vi "Upgrade Firmware (File).vi"(6 "Remote Timeout (300,000 ms)":u32=300000, 7 "Stop Tasks Automatically (T)":bool=TRUE, 8 "error in (no error)":errorcluster, 9 "Always Overwrite (F)":bool, 10 "Firmware File":path, 11 "Resource in":refnum<k20>) -> (0 "error out":errorcluster, 1 "Firmware Status":T1=2 items=["update pending auto restart"=-4, "verifying new image"=-3, "writing/flashing new image"=-2, "waiting for image"=-1, "corrupt firmware, cannot run"=0, "no firmware installed"=1, "normal operation"=2, "update pending user restart"=3, "update pending user action"=4, "update attempt failed"=5], 2 "Detailed Result":string, 3 "Resource out":refnum<k20>)   [LabVIEW 2017, in "nisyscfg.lvlib"]
doc: "Updates the firmware on the target using a firmware file on the local computer."
uses:
  <vilib>/nisyscfg/nisyscfg.lvlib
  <vilib>/nisyscfg/Firmware Status.ctl
  <vilib>/Utility/error.llb/Error Cluster From Error Code.vi
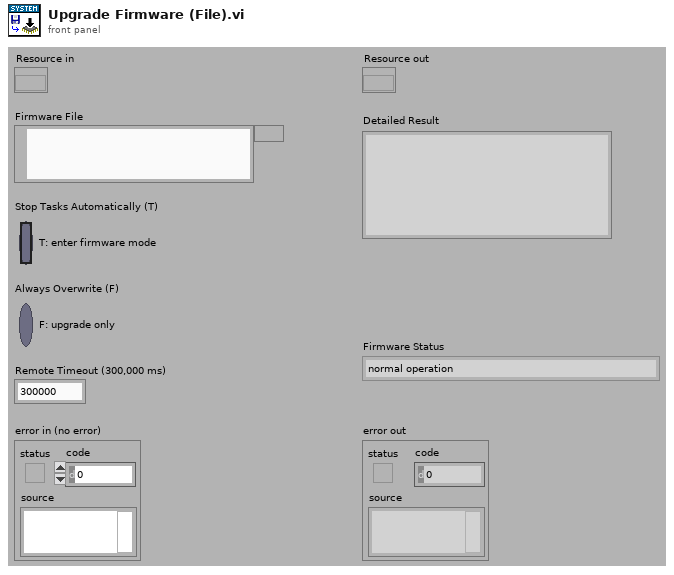
[diagram p1: front panel]
types:
  T1 = typedef "nisyscfg.lvlib/Firmware Status.ctl" = i32
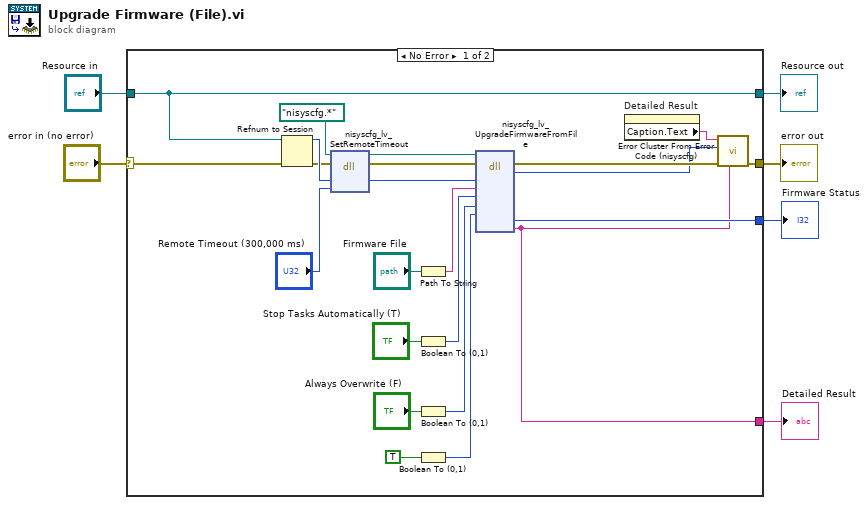
[diagram p0: block diagram]
diagram:
  n1 = case shown="No Error" "error in (no error)" {
    selector: "error in (no error)" -> [w11 w31]
    tunnel: [w29 w31] -> w6
    tunnel: "Resource in" -> [w10 w30]
    tunnel: [w7 _] -> w2
    tunnel: [w10 w30] -> w3
    tunnel: [w9 _] -> w1
    frame No Error {
      n2 = Refnum to Session(4:w11, 7:w10) -> (0:w17:errorcluster, 3:w18:u64)
      n3 = dll-call lib="nisyscfg.*" fn="nisyscfg_lv_SetRemoteTimeout" label="SetRemoteTimeout"(path in=path "nisyscfg.*", error in=w17, "item"=w18, "connectTimeout"="Remote Timeout (300,000 ms)") -> (path out=w12:path, error out=w14:errorcluster, "item"=w13:u64)  [unwired: 1 in, 2 out]
      n4 = Path To String(path="Firmware File") -> (string=w21:string)
      n5 = Boolean To (0,1)(Boolean="Stop Tasks Automatically (T)") -> (0, 1=w25:i16)
      n6 = Boolean To (0,1)(Boolean="Always Overwrite (F)") -> (0, 1=w23:i16)
      n7 = Boolean To (0,1)(Boolean=TRUE) -> (0, 1=w19:i16)
      n8 = dll-call lib="nisyscfg.*" fn="nisyscfg_lv_UpgradeFirmwareFromFile" label="UpgradeFirmwareFromFile"(path in=w12, error in=w14, "itemHandle"=w13, "firmwareFilename"=w21, "stopTasks"=w25, "overwriteIfSameVersion"=w23, "waitForFinish"=w19) -> (error out=w28:errorcluster, "return type"=w27:i32, "firmwareStatus"=w9:i32, "details"=w7:string)  [unwired: 8 in, 1 out]
      n9 = property on="Detailed Result" class="Str"() -> ("Caption.Text"=w8:string)  [unwired: 2 in, 2 out]
      n10 = call <vilib>:"Error Cluster From Error Code (nisyscfg).vi"("Details String"=w7, "error in (no error)"=w28, "Error Code (0)"=w27, "Details Caption"=w8) -> ("error out"=w29:errorcluster)  [unwired: 7 in]
    }
    frame Error {
    }
  }
  "error out" <- w6
  "Resource out" <- w3
  "Firmware Status" <- w1
  "Detailed Result" <- w2
